vi "Get Jacobian.vi"(8 "error in (no error)":errorcluster, 11 "Finger in":refnum<class "Finger.lvclass">) -> (0 "error out":errorcluster, 2 "Jacobian":T1, 3 "Finger out":refnum<class "Finger.lvclass">)   [LabVIEW 2011, in "Finger.lvclass"]
uses:
  Finger.lvclass
  <vilib>/Analysis/Matrix/Datatypes/RealMatrix.ctl
  Finger.lvclass/Finger.ctl
  <vilib>/Analysis/Matrix/Numeric/Multiply/Multiply - RM,RM.vi
  <vilib>/Analysis/Matrix/Numeric/Conversions/Array To Matrix - RA.vi
  <vilib>/Analysis/Matrix/NI_Matrix.lvlib
  <vilib>/robotics/Kinematics/NI_Kinematics.lvlib
  <vilib>/Analysis/NI_AALPro.lvlib
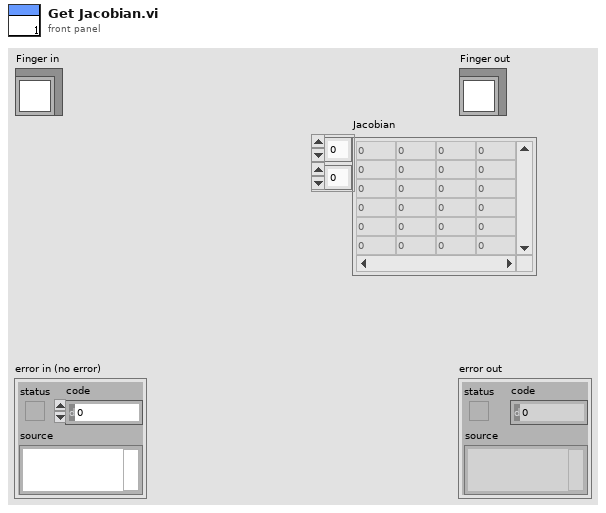
[diagram p1: front panel]
types:
  T1 = typedef "NI_Matrix.lvlib/RealMatrix.ctl" = dbl[][]
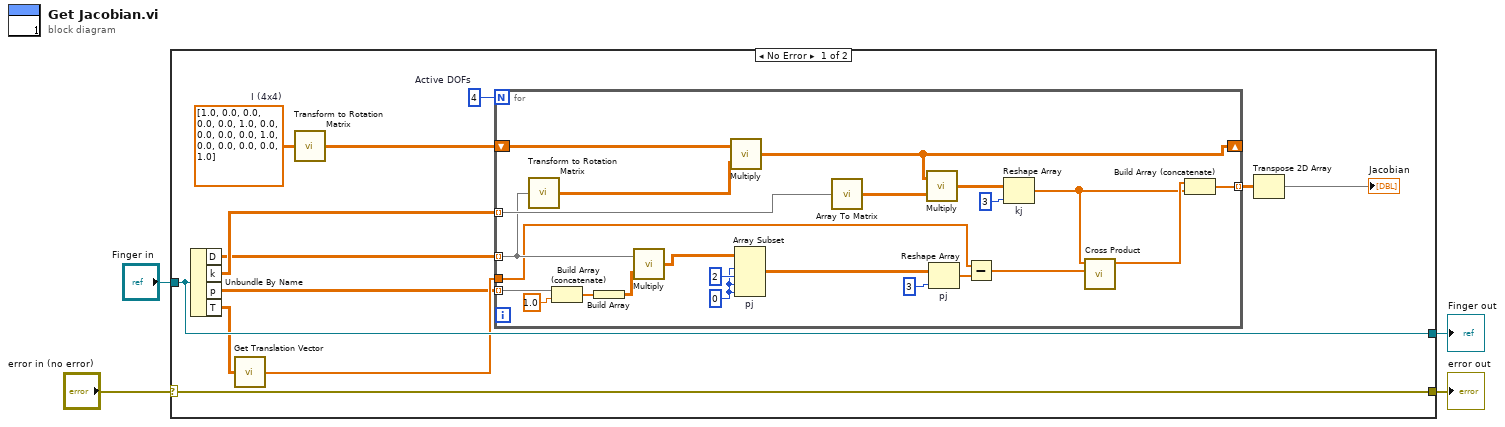
[diagram p0: block diagram]
diagram:
  n1 = case shown="No Error" "error in (no error)" {
    selector: "error in (no error)" -> [w16 w41]
    tunnel: [w16 w41] -> w3
    tunnel: [w15 w40] -> w1
    tunnel: "Finger in" -> [w15 w40]
    frame No Error {
      w14 = 4  # Active DOFs
      w9 = T1 [[1.0, 0.0, 0.0, 0.0], [0.0, 1.0, 0.0, 0.0], [0.0, 0.0, 1.0, 0.0], [0.0, 0.0, 0.0, 1.0]]  # I (4x4)
      n2 = Unbundle By Name(w15) -> ("D"=w6:dbl[][][], "k"=w7:T1, "p"=w8:T1, "T"=w5:T1)
      n3 = call <vilib>:"Get Translation Vector.vi"("transform"=w5) -> ("translation vector"=w12:dbl[])
      n4 = call <vilib>:"Transform to Rotation Matrix.vi"("transform"=w9) -> ("rotation matrix"=w13:T1)
      n5 = for {
        N: w14 -> [_]
        tunnel: w6 -> [w34] mode=indexing
        shift-right: [w37] -> _
        shift-left: w13 -> [w39]
        tunnel: w7 -> [w35] mode=indexing
        tunnel: w8 -> [w19] mode=indexing
        tunnel: w12 -> [w30]
        tunnel: [w21] -> w11 mode=indexing
        w31 = 0 ("row 1")
        n6 = call <vilib>:"Transform to Rotation Matrix.vi"("transform"=w34) -> ("rotation matrix"=w38:T1)
        n7 = Build Array (concatenate)(w19, 1.0) -> (w18:dbl[])
        n8 = Build Array(w18) -> (w20:T1)
        n9 = call-poly <vilib>:"Multiply.vi"("Real Matrix B"=w20, "Real Matrix A"=w34) -> ("A * B"=w33:T1)
        n10 = call-poly <vilib>:"Multiply.vi"("Real Matrix B"=w38, "Real Matrix A"=w39) -> ("A * B"=w37:T1)
        n11 = Array Subset "pj"(array=w33, index (row)=w31, length (row)=2 ("row N"), index (col)=w31, length (col)=w31) -> (w29:T1)
        n12 = call-poly <vilib>:"Array To Matrix.vi"("Real 1D Array"=w35) -> ("Real Matrix (Column Vector)"=w36:T1)
        n13 = call-poly <vilib>:"Multiply.vi"("Real Matrix B"=w36, "Real Matrix A"=w37) -> ("A * B"=w25:T1)
        n14 = Reshape Array "pj"(w29, 3 ("dimension size")) -> (w27:dbl[])
        n15 = Subtract(x=w30, y=w27) -> (x-y=w24:dbl[])
        n16 = Reshape Array "kj"(w25, 3 ("dimension size")) -> (w22:dbl[])
        n17 = call <vilib>:"Cross Product.vi"("B Vector"=w24, "A Vector"=w22) -> ("Cross Product"=w23:dbl[])  [unwired: 8 in, 1 out]
        n18 = Build Array (concatenate)(w23, w22) -> (w21:dbl[])
      }
      n19 = Transpose 2D Array(2D array=w11) -> (transposed array=→"Jacobian":dbl[][])
    }
    frame Error {
    }
  }
  "error out" <- w3
  "Finger out" <- w1
